vi "Vision on New GIC.vi"(11 "GIC Input":T2={"     Use ?\nOff       On"=[FALSE, TRUE, FALSE, TRUE], "Mode:"=FALSE, "WP Data"=0.0, "Hokuyo Port"="COM7", "Prop  Port"="COM6", "Compass Port"="", "GPS Port"="", "Num of WPs"=0, "WP Lats and Longs"={"WP Lats"=[], "WP Longs"=[]}, "Obst Lats and Longs"={"Obst Lats"=[], "Obst Longs"=[]}, "Parameters"=[], "GPS Data"=[], "Compass"=0.0, "LMS Vector"=[], "Vision Vector"=[], "Direction Cmd"=0.0, "Speed Cmd"=0.0, "WP Vector"=[], "WP Number"=0, "Extra"=0, "SW Map"=[], "Path Cluster"={"Path x node"=[], "Path y node"=[]}} {"Obst Lats and Longs"."Obst Longs" format="%#_8g"; "Obst Lats and Longs"."Obst Lats" format="%#_8g"}) -> (3 "GIC Output":T2={"     Use ?\nOff       On"=[FALSE, TRUE, FALSE, TRUE], "Mode:"=FALSE, "WP Data"=0.0, "Hokuyo Port"="COM7", "Prop  Port"="COM6", "Compass Port"="", "GPS Port"="", "Num of WPs"=0, "WP Lats and Longs"={"WP Lats"=[], "WP Longs"=[]}, "Obst Lats and Longs"={"Obst Lats"=[], "Obst Longs"=[]}, "Parameters"=[], "GPS Data"=[], "Compass"=0.0, "LMS Vector"=[], "Vision Vector"=[], "Direction Cmd"=0.0, "Speed Cmd"=0.0, "WP Vector"=[], "WP Number"=0, "Extra"=0, "SW Map"=[], "Path Cluster"={"Path x node"=[], "Path y node"=[]}} {"Obst Lats and Longs"."Obst Longs" format="%#_8g"; "Obst Lats and Longs"."Obst Lats" format="%#_8g"})   [LabVIEW 2014]
panel:
  out "Image Out":T1(plugin-control)
  out "swmap":dbl[][](array[numeric])
  # "Vision on New GIC"
  # "Input:"
  # "Output"
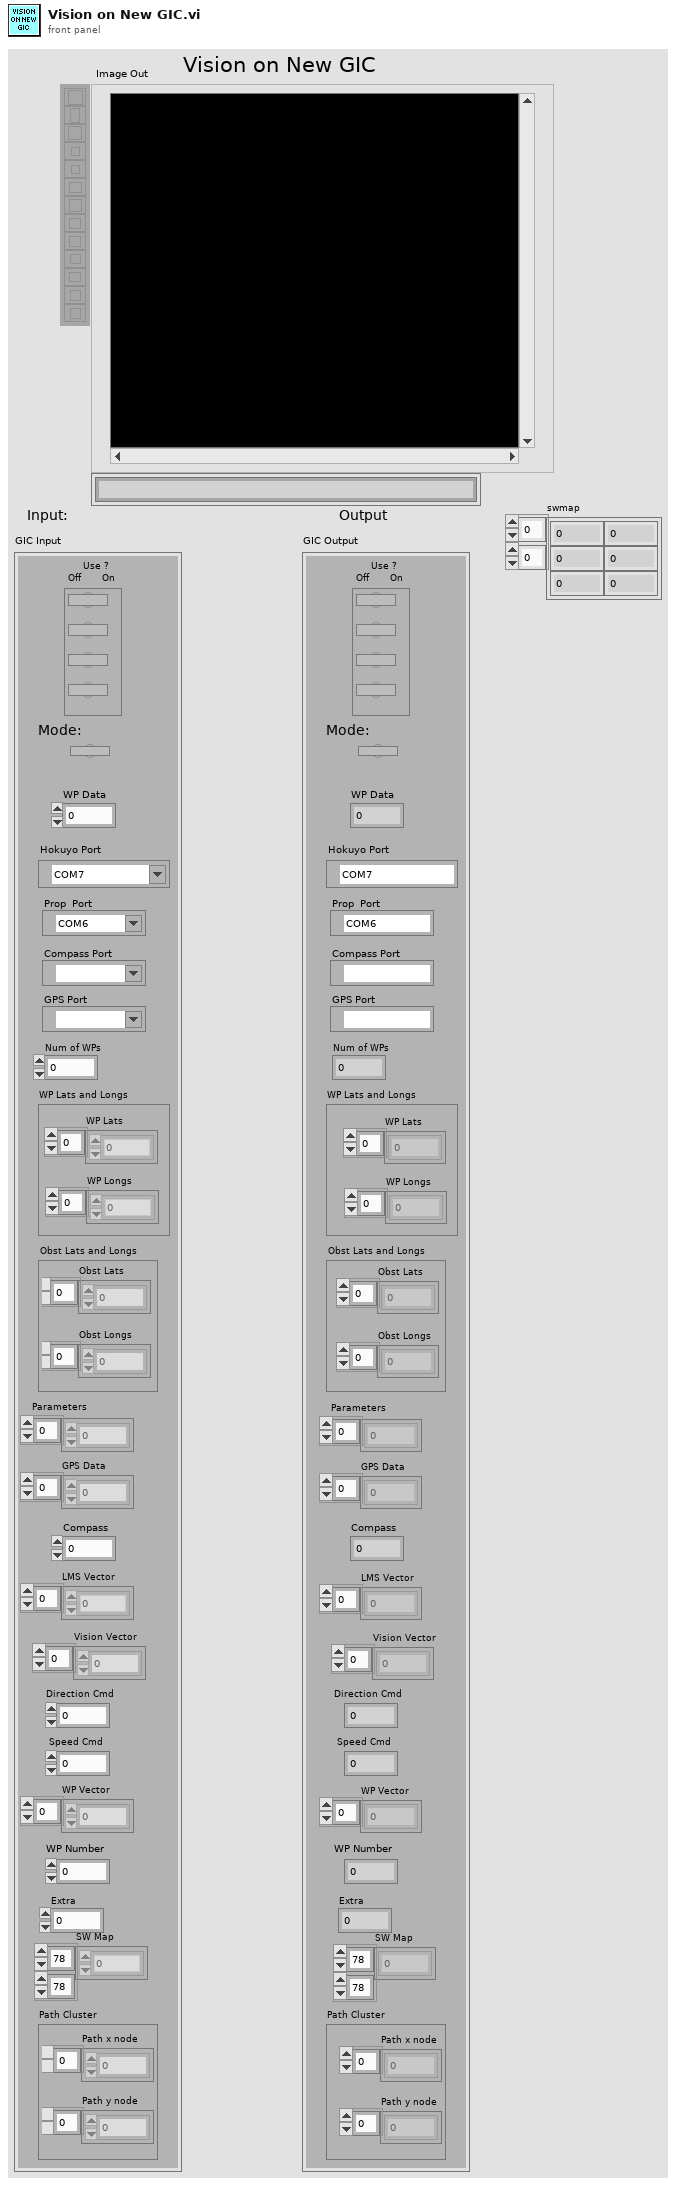
[diagram p1: front panel]
types:
  T1 = typedef "IMAQ Image.ctl" = refnum<image>
  T2 = cluster{"     Use ?\nOff       On":bool[], "Mode:":bool, "WP Data":dbl, "Hokuyo Port":refnum<visa-resource-name>, "Prop  Port":refnum<visa-resource-name>, "Compass Port":refnum<visa-resource-name>, "GPS Port":refnum<visa-resource-name>, "Num of WPs":i16, "WP Lats and Longs":cluster{"WP Lats":dbl[], "WP Longs":dbl[]}, "Obst Lats and Longs":cluster{"Obst Lats":dbl[], "Obst Longs":dbl[]}, "Parameters":dbl[], "GPS Data":dbl[], "Compass":dbl, "LMS Vector":dbl[], "Vision Vector":dbl[], "Direction Cmd":dbl, "Speed Cmd":dbl, "WP Vector":dbl[], "WP Number":i32, "Extra":i16, "SW Map":i32[][], "Path Cluster":cluster{"Path x node":dbl[], "Path y node":dbl[]}}
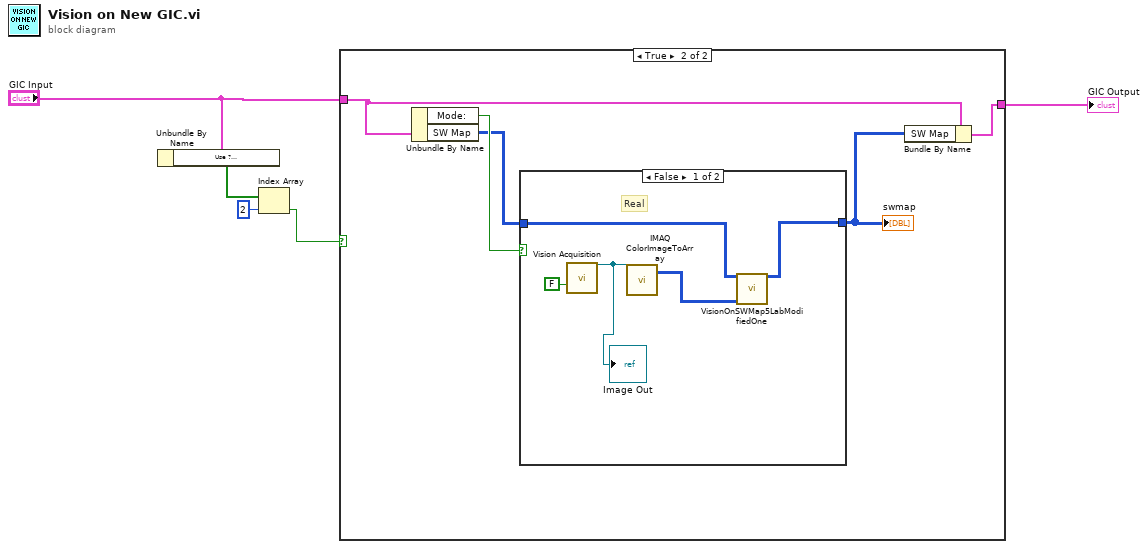
[diagram p0: block diagram]
diagram:
  n1 = Unbundle By Name("GIC Input") -> ("Use ?\nOff       On"=w5:bool[])
  n2 = Index Array(array=w5, index=2) -> (element=w2:bool)
  n3 = case shown="True" w2 {
    tunnel: "GIC Input" -> [w6 w10]
    tunnel: [w6 w8] -> w1
    frame False {
    }
    frame True {
      n4 = Unbundle By Name(w10) -> ("Mode:"=w11:bool, "SW Map"=w7:i32[][])
      n5 = case shown="False" w11 {
        tunnel: w7 -> [w15 w17]
        tunnel: [w13 w17] -> w9
        frame False {
          # "Real"
          n6 = call "Vision Acquisition"("Stop (F)"=FALSE) -> ("Image Out"=w12:T1)  [unwired: 24 in, 2 out]
          "Image Out" <- w12
          n7 = call "IMAQ ColorImageToArray"("Image"=w12) -> ("Image Pixels (U32)"=w16:u32[][])  [unwired: 3 in, 2 out]
          n8 = call "VisionOnSWMap5LabModifiedOne.vi"("SWMap In"=w15, "Image Pixels"=w16) -> ("SWMap Out"=w13:i32[][])  [unwired: 13 in]
        }
        frame True {
          # "Sim"
        }
      }
      "swmap" <- w9
      n9 = Bundle By Name(cluster=w10, "SW Map"=w9) -> (w8:T2)
    }
  }
  "GIC Output" <- w1
